vi "Is_it_a_Results_File.vi"(0 "character string":string) -> (1 "Contain DB Header Info":bool, 2 "Header String":string, 3 "Results File?":bool)   [LabVIEW 2010]
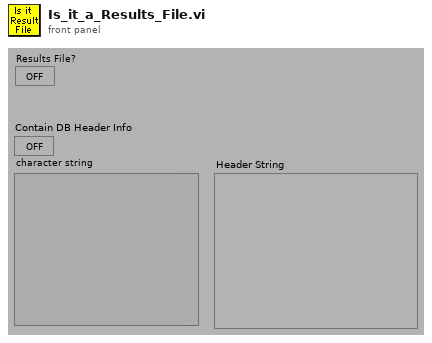
[diagram p1: front panel]
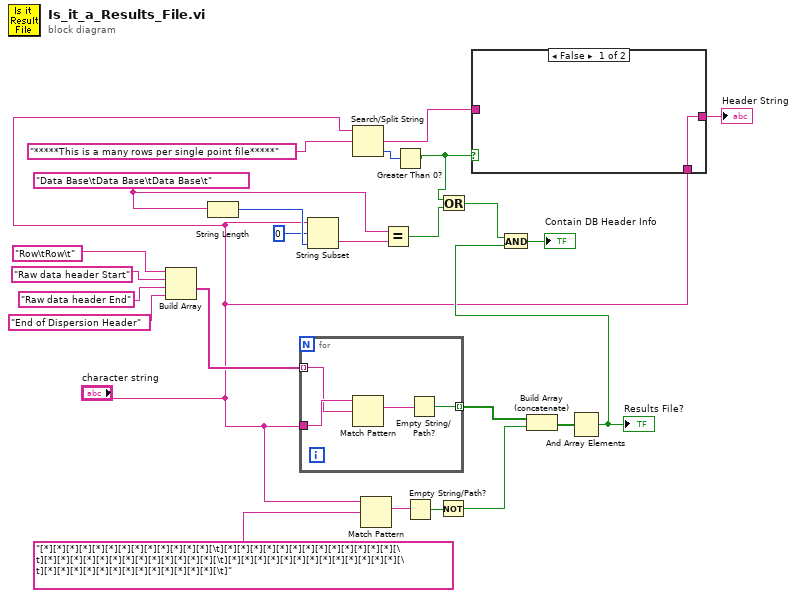
[diagram p0: block diagram]
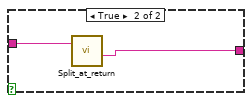
[diagram p2: hidden frame]
diagram:
  w11 = "Data Base\tData Base\tData Base\t"
  n1 = Build Array("Row\tRow\t", "Raw data header Start", "Raw data header End", "End of Dispersion Header") -> (w23:string[])
  n2 = String Length(string=w11) -> (length=w14:i32)
  n3 = for {
    tunnel: "character string" -> [w29]
    tunnel: w23 -> [w28] mode=indexing
    tunnel: [w26] -> w20 mode=indexing
    n4 = Match Pattern(string=w29, regular expression=w28) -> (match substring=w27:string)  [unwired: 4 out]
    n5 = Empty String/Path?(string/path=w27) -> (empty?=w26:bool)
  }
  n6 = String Subset(string="character string", offset (0)=0, length (rest)=w14) -> (substring=w12:string)
  n7 = Search/Split String(string="character string", search string/char (-)="*****This is a many rows per single point file*****") -> (match + rest of string=w6:string, offset of match=w2:i32)  [unwired: 2 out]
  n8 = Match Pattern(string="character string", regular expression="[*][*][*][*][*][*][*][*][*][*][*][*][*][\t][*][*][*][*][*][*][*][*][*][*][*][*][*][\t][*][*][*][*][*][*][*][*][*][*][*][*][*][\t][*][*][*][*][*][*][*][*][*][*][*][*][*][\t][*][*][*][*][*][*][*][*][*][*][*][*][*][\t]" ("String")) -> (match substring=w22:string)  [unwired: 4 out]
  n9 = Equal?(x=w11, y=w12) -> (x = y?=w8:bool)
  n10 = Greater Than 0?(x=w2) -> (x > 0?=w1:bool)
  n11 = Empty String/Path?(string/path=w22) -> (empty?=w21:bool)
  n12 = Not(x=w21) -> (.not. x?=w19:bool)
  n13 = Or(x=w1, y=w8) -> (x .or. y?=w7:bool)
  n14 = case shown="False" w1 {
    tunnel: w6 -> [_ w32]
    tunnel: [w30 w31] -> w5
    tunnel: "character string" -> [w30 _]
    frame False {
    }
    frame True {
      n15 = call "Split_at_return.vi"("String"=w32) -> ("after substring"=w31:string)  [unwired: 1 in, 3 out]
    }
  }
  "Header String" <- w5
  n16 = Build Array (concatenate)(w20, w19) -> (w18:bool[])
  n17 = And Array Elements(Boolean array=w18) -> (logical AND=w10:bool)
  "Results File?" <- w10
  n18 = And(x=w7, y=w10) -> (x .and. y?=→"Contain DB Header Info":bool)
